vi "AutoNameSub.vi"(2 "Time Stamp":timestamp, 3 "Custom Folder":string, 4 "Extention":string="dat", 5 "User Data Folder":path) -> (0 "created path":path, 1 "String":string)   [LabVIEW 2017]
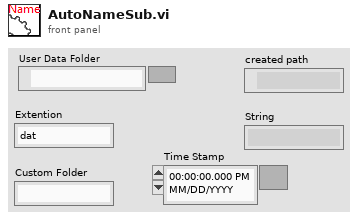
[diagram p1: front panel]
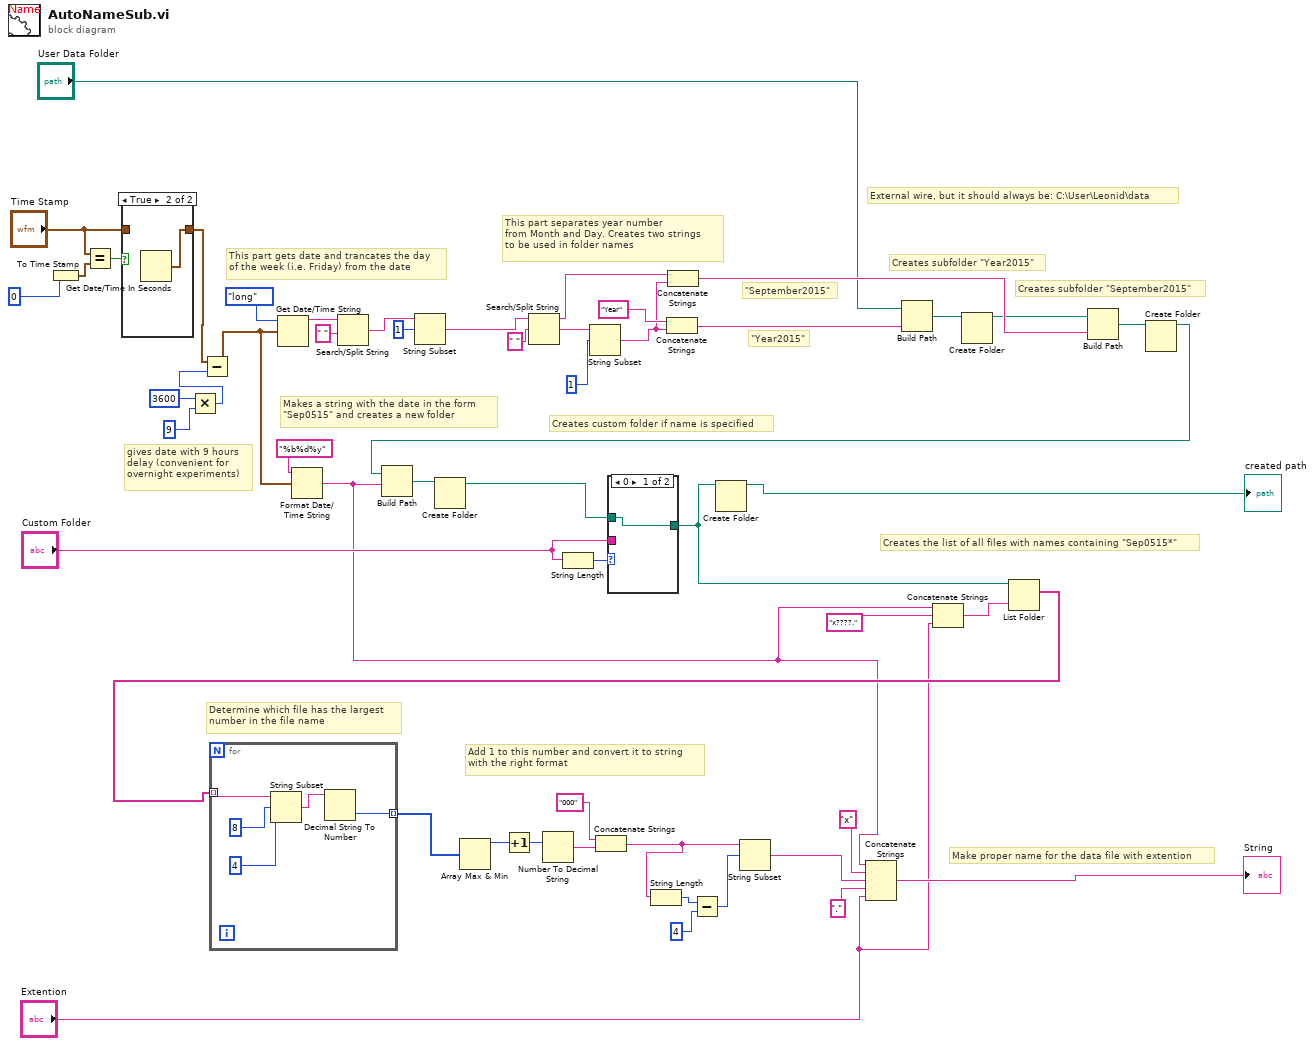
[diagram p0: block diagram]
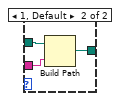
[diagram p3: hidden frame]
diagram:
  # "Add 1 to this number and convert it to string\nwith the right format"
  # "Determine which file has the largest \nnumber in the file name"
  # "External wire, but it should always be: C:\\User\\Leonid\\data"
  # "Make proper name for the data file with extention"
  # "Creates the list of all files with names containing \"Sep0515*\""
  # "Creates custom folder if name is specified"
  # "Makes a string with the date in the form \n\"Sep0515\" and creates a new folder"
  # "Creates subfolder \"September2015\""
  # "Creates subfolder \"Year2015\""
  # "\"September2015\""
  # "\"Year2015\""
  # "This part separates year number \nfrom Month and Day. Creates two strings\nto be used in folder names"
  # "This part gets date and trancates the day \nof the week (i.e. Friday) from the date"
  # "gives date with 9 hours \ndelay (convenient for \novernight experiments)"
  n1 = To Time Stamp(1:0) -> (0:w4:timestamp)
  n2 = Equal?(x="Time Stamp", y=w4) -> (x = y?=w3:bool)
  n3 = case shown="True" w3 {
    tunnel: "Time Stamp" -> [w54 _]
    tunnel: [w54 w55] -> w1
    frame False {
    }
    frame True {
      n4 = Get Date/Time In Seconds() -> (seconds since 1Jan1904=w55:timestamp)
    }
  }
  n5 = Multiply(x=3600, y=9) -> (x*y=w25:i32)
  n6 = Subtract(x=w1, y=w25) -> (x-y=w22:timestamp)
  n7 = Get Date/Time String(date format (0)=enum16{"short", "long", "abbreviated"}."long", seconds (now)=w22) -> (date string=w49:string)  [unwired: 1 in, 1 out]
  n8 = Format Date/Time String(time format string (%c)="%b%d%y", seconds (now)=w22) -> (date/time string=w8:string)  [unwired: 1 in]
  n9 = Search/Split String(string=w49, search string/char (-)=" ") -> (match + rest of string=w47:string)  [unwired: 1 in, 2 out]
  n10 = String Subset(string=w47, offset (0)=1) -> (substring=w42:string)  [unwired: 1 in]
  n11 = Search/Split String(string=w42, search string/char (-)=" ") -> (substring before match=w38:string, match + rest of string=w43:string)  [unwired: 1 in, 1 out]
  n12 = String Length(string="Custom Folder") -> (length=w24:i32)
  n13 = String Subset(string=w43, offset (0)=1) -> (substring=w39:string)  [unwired: 1 in]
  n14 = Concatenate Strings("Year" ("Substring"), w39) -> (w40:string)
  n15 = Concatenate Strings(w38, w39) -> (w37:string)
  n16 = Build Path(base path="User Data Folder", name or relative path=w40) -> (appended path=w36:path)
  n17 = Concatenate Strings(w8, "x????.", "Extention") -> (w52:string)
  n18 = Create Folder(path (use dialog)=w36) -> (created path=w35:path)  [unwired: 2 in, 2 out]
  n19 = Build Path(base path=w35, name or relative path=w37) -> (appended path=w34:path)
  n20 = Create Folder(path (use dialog)=w34) -> (created path=w33:path)  [unwired: 2 in, 2 out]
  n21 = Build Path(base path=w33, name or relative path=w8) -> (appended path=w28:path)
  n22 = Create Folder(path (use dialog)=w28) -> (created path=w29:path)  [unwired: 2 in, 2 out]
  n23 = case shown="0" w24 {
    tunnel: [w56 w59] -> w30
    tunnel: w29 -> [w56 w58]
    tunnel: "Custom Folder" -> [_ w57]
    frame 0 {
    }
    frame 1, Default {
      n24 = Build Path(base path=w58, name or relative path=w57) -> (appended path=w59:path)
    }
  }
  n25 = Create Folder(path (use dialog)=w30) -> (created path=→"created path":path)  [unwired: 2 in, 2 out]
  n26 = List Folder(path=w30, pattern=w52) -> (filenames=w21:string[])  [unwired: 2 in, 3 out]
  n27 = for {
    tunnel: w21 -> [w64] mode=indexing
    tunnel: [w60] -> w20 mode=indexing
    n28 = String Subset(string=w64, offset (0)=8, length (rest)=4) -> (substring=w61:string)
    n29 = Decimal String To Number(string=w61) -> (number=w60:i32)  [unwired: 2 in, 1 out]
  }
  n30 = Array Max & Min(array=w20) -> (max value=w19:i32)  [unwired: 3 out]
  n31 = Increment(x=w19) -> (x+1=w18:i32)
  n32 = Number To Decimal String(number=w18) -> (decimal integer string=w17:string)  [unwired: 1 in]
  n33 = Concatenate Strings("000", w17) -> (w12:string)
  n34 = String Length(string=w12) -> (length=w15:i32)
  n35 = Subtract(x=w15, y=4) -> (x-y=w13:i32)
  n36 = String Subset(string=w12, offset (0)=w13) -> (substring=w9:string)  [unwired: 1 in]
  n37 = Concatenate Strings(w8, "x", w9, "." ("Substring"), "Extention") -> (→"String":string)
